vi "Case Structure.vi"() -> ()   [LabVIEW 2021]
panel:
  in  "PB":bool
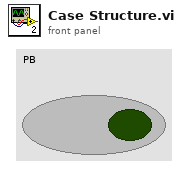
[diagram p1: front panel]
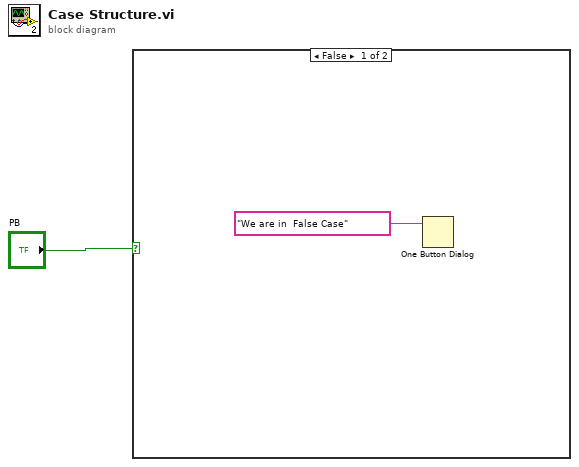
[diagram p0: block diagram]
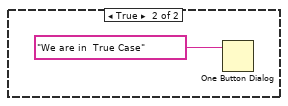
[diagram p2: hidden frame]
diagram:
  n1 = case shown="False" "PB" {
    frame False {
      n2 = One Button Dialog(message="We are in  False Case") -> ()  [unwired: 1 in, 1 out]
    }
    frame True {
      n3 = One Button Dialog(message="We are in  True Case") -> ()  [unwired: 1 in, 1 out]
    }
  }
